vi "VI Server_Get Menu Ring Selection.vi"(7 "Label":string, 8 "error in":errorcluster, 9 "Single Instance (T)":bool=TRUE, 11 "VI Server Cluster":T1) -> (0 "error out":errorcluster, 1 "Control Reference":refnum<vi>, 2 "Selection":string, 3 "VI Server Cluster.DUP":T1, 4 "Value":u16, 6 "Label.Text":string)   [LabVIEW 2020, in "VI Server Toolkit LV2013.lvlib"]
doc: "Returns Item Name selected of the Menu Ring."
uses:
  VI Server Toolkit LV2013.lvlib
  VI Server_TypeDefs/VI Server_RefsCluster.ctl
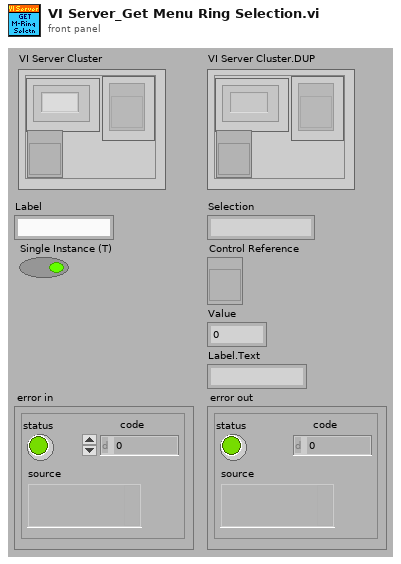
[diagram p1: front panel]
types:
  T1 = typedef "VI Server_RefsCluster.ctl" = cluster{"Labels":string[], "Refs":refnum<vi>[], "VI Ref":refnum<vi>}
  T2 = typedef "LVStringsAndValuesArrayTypeDef_U16.ctl" = cluster{"String":string, "Value":u16}[]
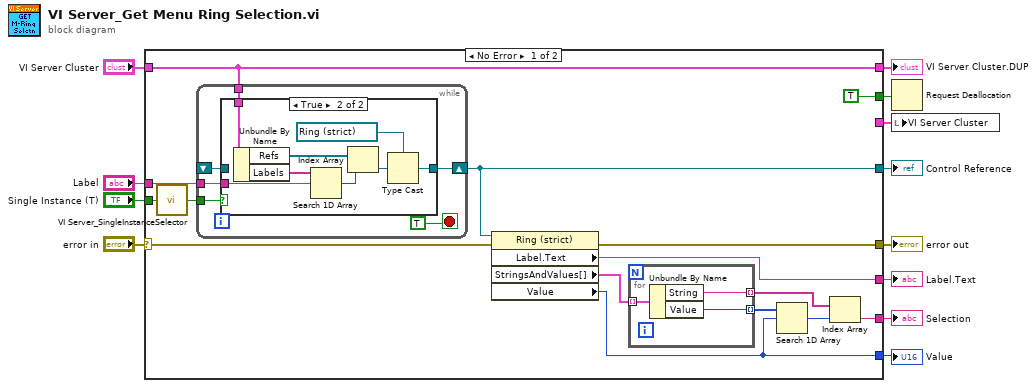
[diagram p0: block diagram]
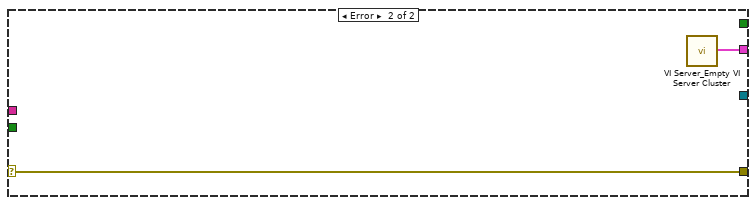
[diagram p3: hidden frame]
diagram:
  n1 = case shown="No Error" "error in" {
    selector: "error in" -> [w26 w47]
    tunnel: "Label" -> [w27 _]
    tunnel: "VI Server Cluster" -> [w23 _]
    tunnel: [w25 w47] -> w12
    tunnel: [w13 _] -> w8
    tunnel: [w18 _] -> w7
    tunnel: [w17 _] -> w6
    tunnel: [w24 _] -> w5
    tunnel: [w23 _] -> w4
    tunnel: [TRUE _] -> w3
    tunnel: [_ w46] -> w2
    tunnel: "Single Instance (T)" -> [w14 _]
    frame No Error {
      n2 = call "VI Server_SingleInstanceSelector.vi"("Single Instance (T)"=w14) -> ("Single Instance.OUT"=w15:bool)  [unwired: 6 in]
      n3 = while {
        tunnel: w27 -> [w33]
        tunnel: w23 -> [w32]
        tunnel: w15 -> [w31]
        shift-right: [w30] -> w13
        shift-left: _ -> [w29]
        stop <- TRUE stop-if-true
        n4 = case shown="True" w31 {
          tunnel: w33 -> [_ w41]
          tunnel: [w34 w37] -> w30
          tunnel: w32 -> [_ w36]
          tunnel: w29 -> [w34 _]
          frame False {
          }
          frame True {
            n5 = Unbundle By Name(w36) -> ("Refs"=w39:refnum<vi>[], "Labels"=w42:string[])
            n6 = Search 1D Array(1D array=w42, element=w41) -> (index of element=w40:i32)  [unwired: 1 out]
            n7 = Index Array(array=w39, index=w40) -> (element=w38:refnum<vi>)
            n8 = Type Cast(type=refnum<vi> refnum ("Ring"), x=w38) -> (*(type *) &x=w37:refnum<vi>)
          }
        }
      }
      n9 = property class="Ring (strict)"(reference=w13, error in=w26) -> (error out=w25:errorcluster, "Label.Text"=w24:string, "StringsAndValues[]"=w22:T2, "Value"=w17:u16)  [unwired: 1 out]
      n10 = for {
        tunnel: w22 -> [w45] mode=indexing
        tunnel: [w44] -> w21 mode=indexing
        tunnel: [w43] -> w19 mode=indexing
        n11 = Unbundle By Name(w45) -> ("String"=w43:string, "Value"=w44:u16)
      }
      n12 = Search 1D Array(1D array=w21, element=w17) -> (index of element=w20:i32)  [unwired: 1 in]
      n13 = Index Array(array=w19, index=w20) -> (element=w18:string)
    }
    frame Error {
      n14 = call "VI Server_Empty VI Server Cluster.vi"() -> ("VI Server Cluster"=w46:T1)  [unwired: 7 in]
    }
  }
  "error out" <- w12
  "VI Server Cluster.DUP" <- w4
  "Control Reference" <- w8
  "Selection" <- w7
  "Value" <- w6
  "Label.Text" <- w5
  n15 = Request Deallocation(w3) -> ()
  n16 = local write "VI Server Cluster"(w2) -> ()
